vi "Polish BD Constant.vi"(10 "BD Const":refnum<vi>, 11 "Identity Writer in":refnum<class "Identity Writer.lvclass">) -> (3 "Identity Writer out":refnum<class "Identity Writer.lvclass">)   [LabVIEW 2013, in "Identity Writer.lvclass"]
doc: "Copyright (c) 2016 Sze Howe Koh\n\nThis Source Code Form is subject to the terms of the Mozilla Public License, v. 2.0. If a copy of the MPL was not distributed with this file, You can obtain one at http://mozilla.org/MPL/2.0/."
uses:
  Identity Writer.lvclass
  <vilib>/numeric/LVNumericRepresentation.ctl
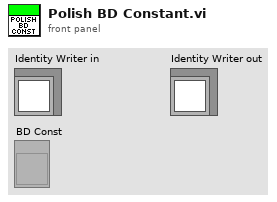
[diagram p1: front panel]
types:
  T1 = typedef "LVNumericRepresentation.ctl" = enum32{"Extended Precision", "Double Precision", "Single Precision", "Long", "Word", "Byte", "Unsigned Long", "Unsigned Word", "Unsigned Byte", "Complex Extended", "Complex Double", "Complex Single", "Quad", "Unsigned Quad", "Fixed-Point"}
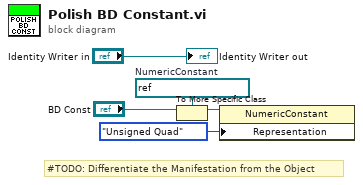
[diagram p0: block diagram]
diagram:
  w4 = refnum<vi> refnum  # NumericConstant
  # "#TODO: Differentiate the Manifestation from the Object"
  n1 = To More Specific Class(target class=w4, reference="BD Const") -> (specific class reference=w3:refnum<vi>)  [unwired: 1 in, 1 out]
  n2 = property class="NumericConstant"(reference=w3, "Representation"=LVNumericRepresentation."Unsigned Quad") -> ()  [unwired: 1 in, 2 out]
  "Identity Writer out" <- "Identity Writer in"
